vi "Drive Controller.vi"(8 "error in":errorcluster) -> ()   [LabVIEW 2017]
doc: "This VI executes continuously carrying out the current operation and responding to updates or new operation requests. It will often contain the timing or control code that is difficult to place directly in TeleOp. This VI generally opens all sensors and motors and isolates the rest of the robot code from knowing implementation details of how the operations are carried out."
uses:
  <vilib>/Rock Robotics/WPI/Framework/Completion Status.ctl
  Drive Setpoints.ctl
  Drive Operations.ctl
  <vilib>/Rock Robotics/WPI/SafetyOutput/WPI_SafetyOutputConfigMenu.ctl
  Phoenix-LabVIEW/Motor Controller/Controls/CTRE_Phoenix_MotorControl_FeedbackDevice.ctl
  Phoenix-LabVIEW/Motor Controller/Controls/CTRE_Phoenix_MotorControl_NeutralMode.ctl
  Drive Published Globals.vi
  <vilib>/Rock Robotics/WPI/RobotDrive/WPI_RobotDriveOpen2MotorWithExistingMotors.vi
  Framework/Robot Global Data.vi
  Phoenix-LabVIEW/Motor Controller/Get/CTRE_Phoenix_MotorController_GetQuadratureData.vi
  <vilib>/Rock Robotics/WPI/RobotDrive/WPI_RobotDriveArcadeDrive_Standard(NoSaturation).vi
  <vilib>/Rock Robotics/Network Tables/NT Write Numeric Array.vi
panel:
  out "RDriveEncoder 2":i32
  out "LDriveEncoder 2":i32
  out "UseLDriveEncoder 2":bool
  out "TargetEncValue":dbl
  out "DegreesToTravel":dbl
  out "UseLDriveEncoder":bool
  out "LDriveEncoder":i32
  out "RDriveEncoder":i32
  out "DriveLastCommandStatus":T1
  in  "Interactive Values":T2
  in  "Buttons":cluster{"Execute Cmd":bool, "Abort Cmd":bool}
  out "Command Timing":cluster{"Start Time (ms)":u32, "Iterations":i32}
  out "Status":T1
  out "Setpoints":T4(graph)
  out "Current\nCmd":string
  # "Tip: The graph shows the motor setpoints. It may also be helpful to observe inputs and sensor values.  You may also want to display tuning or debugging controls."
  # "Interactive Command: You may fill in the settings for a command\nand schedule it with the Execute button. You can observe and abort\nany command while fine tuning the code for the controller."
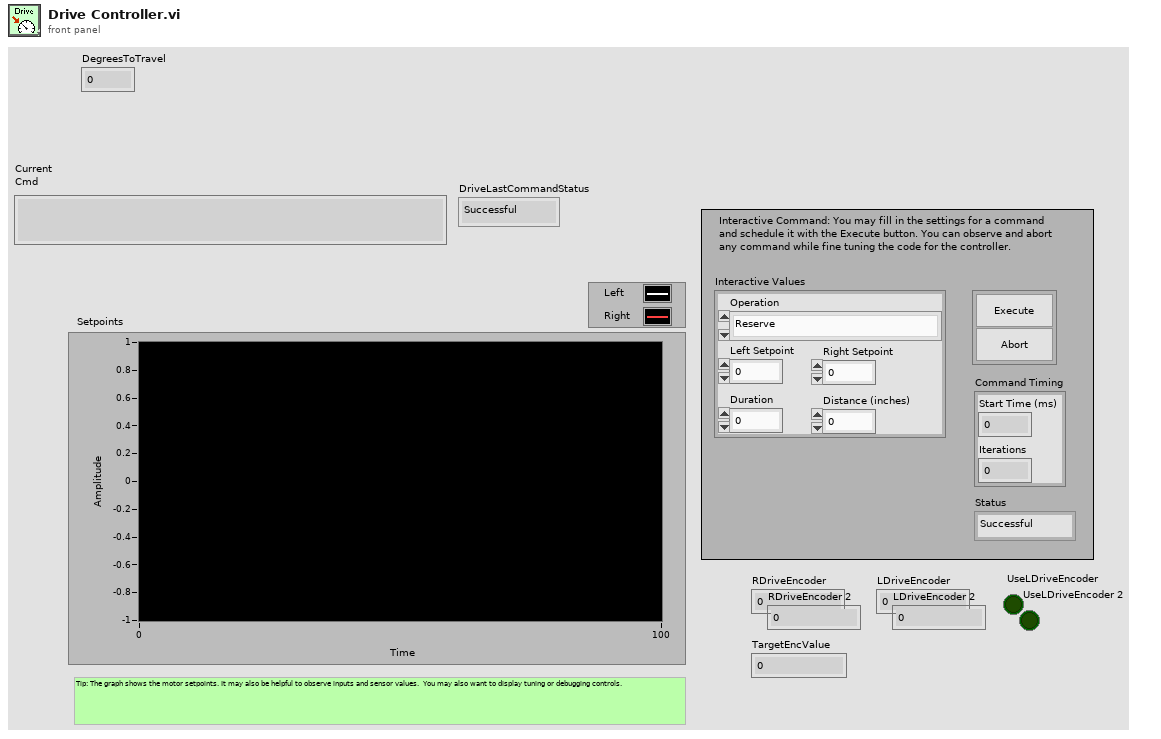
[diagram p1: front panel]
types:
  T1 = typedef "Completion Status.ctl" = enum16{"Successful", "Aborted", "Incomplete"}
  T2 = typedef "Drive Setpoints.ctl" = cluster{"Operation":T3, "Left Setpoint":dbl, "Right Setpoint":dbl, "Duration":dbl, "Distance (inches)":dbl}
  T3 = typedef "Drive Operations.ctl" = enum16{"Reserve", "Read Current", "Immediate", "Drive for Time", "Drive for Distance", "Rotate"}
  T4 = cluster{"Left Setpoint":dbl, "Right Setpoint":dbl}
  T5 = typedef "WPI_SafetyOutputConfigMenu.ctl" = enum16{"Enable", "Disable"}
  T6 = typedef "CTRE_Phoenix_MotorControl_FeedbackDevice.ctl" = i8
  T7 = typedef "WPI_MotorControlDeviceRef.ctl" = cluster{"DeviceStatus":errorcluster, "Type":T8, "PWM":cluster{"PWM Channel":T9, "DeadBand":T10}, "CAN":cluster{"Device Number":u8, "SetOutput VI Ref":variant, "GetOutput VI Ref":variant, "Enable VI Ref":variant, "Disable VI Ref":variant, "Data":variant}, "Invert":bool, "DIO PWM":cluster{"PWM \"Enable\" Channel":T9, "DIOChannel":T11, "PWM Rate":dbl}}
  T8 = typedef "WPI_MotorControlType.ctl" = enum16{"PWM", "CAN", "DIO PWM"}
  T9 = typedef "FPGA_DIOPWMChannel.ctl" = enum8{"PWM 0", "PWM 1", "PWM 2", "PWM 3", "PWM 4", "PWM 5", "PWM 6", "PWM 7", "PWM 8", "PWM 9", "PWM MXP 0", "PWM MXP 1", "PWM MXP 2", "PWM MXP 3", "PWM MXP 4", "PWM MXP 5", "PWM MXP 6", "PWM MXP 7", "PWM MXP 8", "PWM MXP 9", "Invalid"}
  T10 = typedef "WPI_PWMDeadband.ctl" = cluster{"Name":string, "maxPositivePwm":i32, "minPositivePwm":i32, "centerPwm":i32, "maxNegativePwm":i32, "minNegativePwm":i32, "angularRange":u16}
  T11 = typedef "FPGA_DIOChannel.ctl" = enum8{"DIO 0", "DIO 1", "DIO 2", "DIO 3", "DIO 4", "DIO 5", "DIO 6", "DIO 7", "DIO 8", "DIO 9", "DIO MXP 0", "DIO MXP 1", "DIO MXP 2", "DIO MXP 3", "DIO MXP 4", "DIO MXP 5", "DIO MXP 6", "DIO MXP 7", "DIO MXP 8", "DIO MXP 9", "DIO MXP 10", "DIO MXP 11", "DIO MXP 12", "DIO MXP 13", "DIO MXP 14", "DIO MXP 15", "SPI Port CS1", "SPI Port CS2", "SPI Port CS3", "SPI Port MISO", "SPI Port MOSI", "Invalid"}
  T12 = typedef "WPI_RobotDriveDevRef.ctl" = cluster{"DevStatus":errorcluster, "Motors[]":T7[], "Square Inputs":bool, "Max Output":dbl}
  T13 = typedef "Command Status Info.ctl" = cluster{"Name":string, "Status":T1, "notifier out":T14}
  T14 = typedef "Completion Notifier.ctl" = refnum<notifier>
  T15 = cluster{"SubSystem Data":T2, cluster{"Start Time (ms)":u32, "Iterations":i32}, cluster{"Command Info":T13, "Description":string, "Default Command":T2, "queue out":refnum<queue>, "Subsystem Name":string}}
  T16 = typedef "CTRE_Phoenix_MotorControl_NeutralMode.ctl" = enum8{"EEPROMSetting", "Override to Coast", "Override to Brake"}
  T17 = cluster{"SubSystem Data":T2, cluster{"Start Time (ms)":u32, "Iterations":i32}, "Default Command Arguments":cluster{"Command Info":T13, "Description":string, "Default Command":T2, "queue out":refnum<queue>, "Subsystem Name":string}}
  T18 = cluster{"Don't move motors while reserved":dbl, "Don't move motors while reserved":dbl}
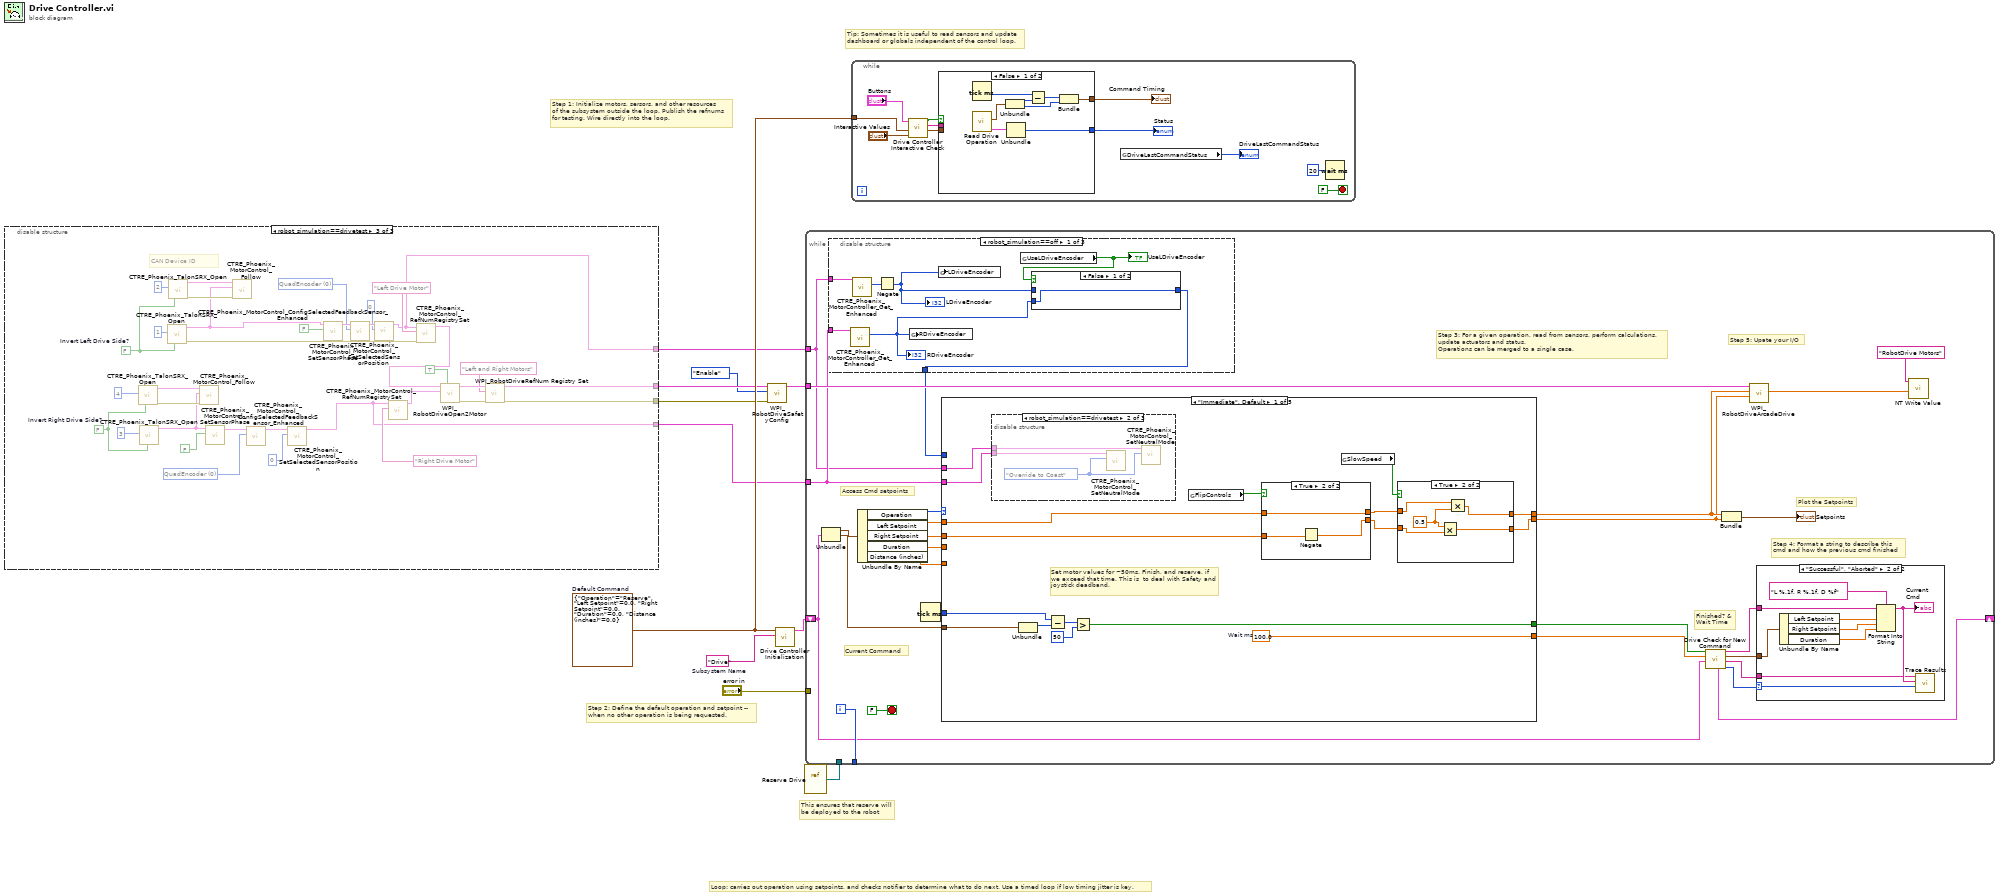
[diagram p0: block diagram]
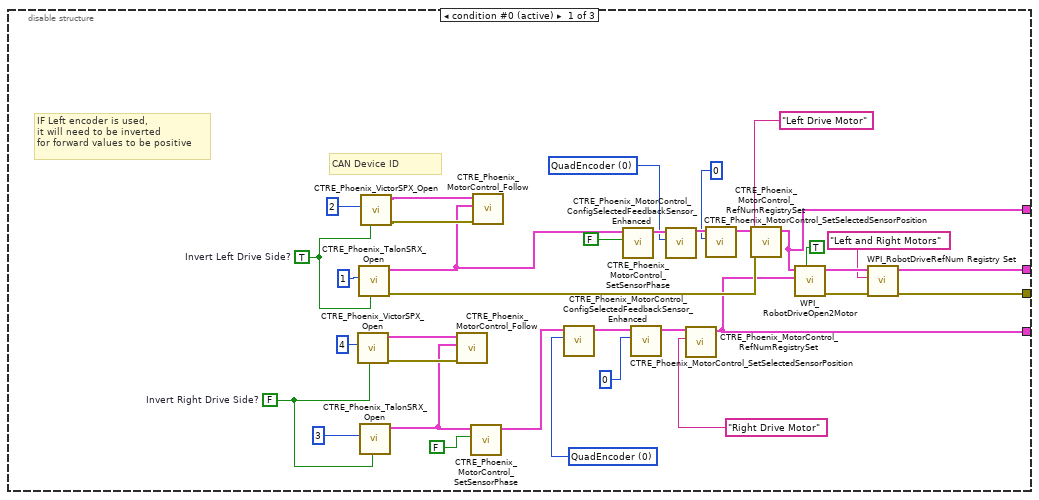
[diagram p2: hidden frame]
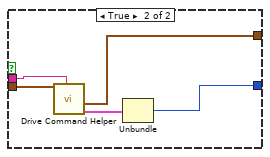
[diagram p4: hidden frame]
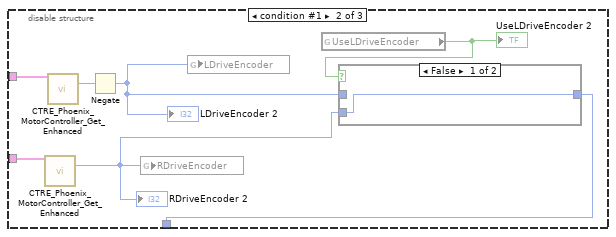
[diagram p6: hidden frame]
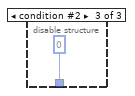
[diagram p8: hidden frame]
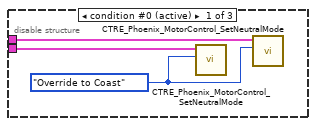
[diagram p11: hidden frame]
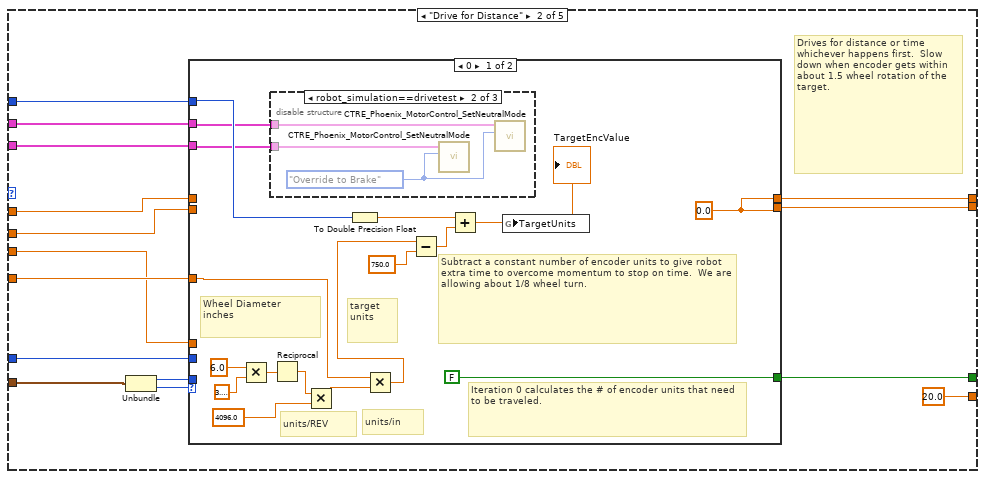
[diagram p14: hidden frame]
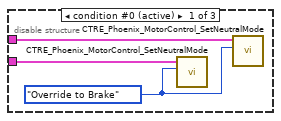
[diagram p15: hidden frame]
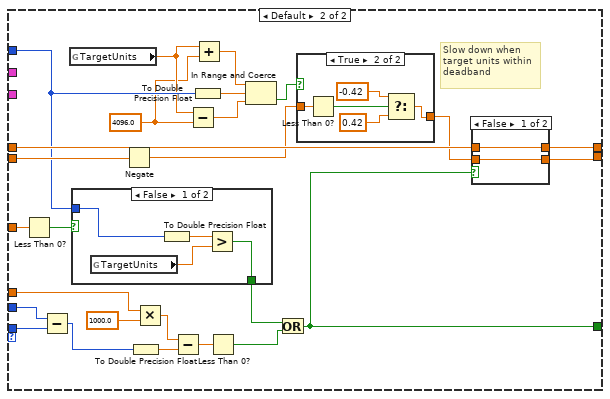
[diagram p17: hidden frame]
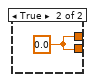
[diagram p19: hidden frame]
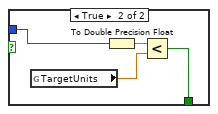
[diagram p20: hidden frame]
diagram:
  w6 = T2 {"Operation"=enum."Reserve", "Left Setpoint"=0.0, "Right Setpoint"=0.0, "Duration"=0.0, "Distance (inches)"=0.0}  # Default Command
  w11 = "Drive"  # Subsystem Name
  # "This ensures that reserve will\nbe deployed to the robot"
  # "Tip: Sometimes it is useful to read sensors and update\ndashboard or globals independent of the control loop."
  # "Step 2: Define the default operation and setpoint --\nwhen no other operation is being requested."
  # "Step 1: Initialize motors, sersors, and other resources\nof the subsystem outside the loop. Publish the refnums\nfor testing. Wire directly into the loop."
  # "Loop: carries out operation using setpoints, and checks notifier to determine what to do next. Use a timed loop if low timing jitter is key."
  n1 = disable-structure shown="robot_simulation==drivetest" {
    disable-tunnel: [w39 _ w64] -> w5
    disable-tunnel: [w38 _ w63] -> w4
    disable-tunnel: [w21 _ w49] -> w2
    disable-tunnel: [w15 _ w50] -> w1
    frame condition #0 (active) {
      w17 = T6 0 items=["None"=-1, "QuadEncoder"=0, "Analog"=2, "Tachometer"=4, "Pulse Width Encoded Position"=8, "Sensor Sum (S0 + S1)"=9, "Sensor Difference (D0 - D1)"=10, "Remote Source 0"=11, "Remote Source 1"=12, "Software Emulated"=15] ("Feedback Device")
      w26 = T6 0 items=["None"=-1, "QuadEncoder"=0, "Analog"=2, "Tachometer"=4, "Pulse Width Encoded Position"=8, "Sensor Sum (S0 + S1)"=9, "Sensor Difference (D0 - D1)"=10, "Remote Source 0"=11, "Remote Source 1"=12, "Software Emulated"=15] ("Feedback Device")
      w32 = TRUE  # Invert Left Drive Side?
      w30 = FALSE  # Invert Right Drive Side?
      # "IF Left encoder is used,\nit will need to be inverted\nfor forward values to be positive"
      # "CAN Device ID"
      n2 = call "CTRE_Phoenix_VictorSPX_Open.vi"("Invert"=w30, "Device Number"=u8 4) -> ("error out"=w41:errorcluster, "CAN Talon SRX Ref"=w40:T7)  [unwired: 8 in]
      n3 = call "CTRE_Phoenix_TalonSRX_Open.vi"("Invert"=w32, "Device Number"=u8 1) -> ("error out"=w42:errorcluster, "CAN Talon SRX Ref"=w13:T7)  [unwired: 8 in]
      n4 = call "CTRE_Phoenix_TalonSRX_Open.vi"("Invert"=w30, "Device Number"=u8 3) -> ("CAN Talon SRX Ref"=w28:T7)  [unwired: 8 in, 1 out]
      n5 = call "CTRE_Phoenix_VictorSPX_Open.vi"("Invert"=w32, "Device Number"=u8 2) -> ("error out"=w35:errorcluster, "CAN Talon SRX Ref"=w36:T7)  [unwired: 8 in]
      n6 = call "CTRE_Phoenix_MotorControl_Follow.vi"("error in (no error)"=w41, "Master Controller to Follow"=w28, "PhoenixMotorControlDevRef"=w40) -> ()  [unwired: 7 in, 2 out]
      n7 = call "CTRE_Phoenix_MotorControl_SetSensorPhase.vi"("PhaseSensor"=FALSE, "PhoenixMotorControlDevRef"=w28) -> ("PhoenixMotorControlDevRef"=w24:T7)  [unwired: 8 in, 1 out]
      n8 = call "CTRE_Phoenix_MotorControl_Follow.vi"("error in (no error)"=w35, "Master Controller to Follow"=w13, "PhoenixMotorControlDevRef"=w36) -> ()  [unwired: 7 in, 2 out]
      n9 = call "CTRE_Phoenix_MotorControl_ConfigSelectedFeedbackSensor_Enhanced.vi"("Feedback Device"=w26, "PhoenixMotorControlDevRef"=w24) -> ("PhoenixMotorControlDevRef"=w23:T7)  [unwired: 8 in, 1 out]
      n10 = call "CTRE_Phoenix_MotorControl_SetSensorPhase.vi"("PhaseSensor"=FALSE, "PhoenixMotorControlDevRef"=w13) -> ("PhoenixMotorControlDevRef"=w19:T7)  [unwired: 8 in, 1 out]
      n11 = call "CTRE_Phoenix_MotorControl_SetSelectedSensorPosition.vi"("New Sensor Position"=0, "PhoenixMotorControlDevRef"=w23) -> ("PhoenixMotorControlDevRef"=w22:T7)  [unwired: 8 in, 1 out]
      n12 = call "CTRE_Phoenix_MotorControl_ConfigSelectedFeedbackSensor_Enhanced.vi"("Feedback Device"=w17, "PhoenixMotorControlDevRef"=w19) -> ("PhoenixMotorControlDevRef"=w20:T7)  [unwired: 8 in, 1 out]
      n13 = call "CTRE_Phoenix_MotorControl_RefNumRegistrySet.vi"("refnum name"="Right Drive Motor", "PhoenixMotorControlDevRef"=w22) -> ("PhoenixMotorControlDevRef"=w21:T7)  [unwired: 8 in, 1 out]
      n14 = call "CTRE_Phoenix_MotorControl_SetSelectedSensorPosition.vi"("New Sensor Position"=0, "PhoenixMotorControlDevRef"=w20) -> ("PhoenixMotorControlDevRef"=w14:T7)  [unwired: 8 in, 1 out]
      n15 = call "CTRE_Phoenix_MotorControl_RefNumRegistrySet.vi"("error in (no error)"=w42, "refnum name"="Left Drive Motor", "PhoenixMotorControlDevRef"=w14) -> ("PhoenixMotorControlDevRef"=w15:T7)  [unwired: 7 in, 1 out]
      n16 = call-poly <vilib>:"WPI_RobotDriveOpen2Motor.vi"("Square Inputs"=TRUE, "Right Motor Dev Ref"=w21, "Left Motor Dev Ref"=w15) -> ("error out"=w44:errorcluster, "RobotDriveDevRef"=w46:T12)  [unwired: 2 in, 5 out]
      n17 = call <vilib>:"WPI_RobotDriveRefNum Registry Set.vi"("error in (no error)"=w44, "refnum name"="Left and Right Motors", "RobotDriveDevRef"=w46) -> ("error out"=w38:errorcluster, "RobotDriveDevRef"=w39:T12)  [unwired: 1 in, 6 out]
    }
    frame condition #1 {
    }
    frame condition #2 {
      w52 = T6 0 items=["None"=-1, "QuadEncoder"=0, "Analog"=2, "Tachometer"=4, "Pulse Width Encoded Position"=8, "Sensor Sum (S0 + S1)"=9, "Sensor Difference (D0 - D1)"=10, "Remote Source 0"=11, "Remote Source 1"=12, "Software Emulated"=15] ("Feedback Device")
      w56 = T6 0 items=["None"=-1, "QuadEncoder"=0, "Analog"=2, "Tachometer"=4, "Pulse Width Encoded Position"=8, "Sensor Sum (S0 + S1)"=9, "Sensor Difference (D0 - D1)"=10, "Remote Source 0"=11, "Remote Source 1"=12, "Software Emulated"=15] ("Feedback Device")
      w71 = FALSE  # Invert Left Drive Side?
      w62 = FALSE  # Invert Right Drive Side?
      # "CAN Device ID"
      n18 = call "CTRE_Phoenix_TalonSRX_Open.vi"("Invert"=w62, "Device Number"=u8 4) -> ("error out"=w74:errorcluster, "CAN Talon SRX Ref"=w73:T7)  [unwired: 8 in]
      n19 = call "CTRE_Phoenix_TalonSRX_Open.vi"("Invert"=w62, "Device Number"=u8 3) -> ("CAN Talon SRX Ref"=w61:T7)  [unwired: 8 in, 1 out]
      n20 = call "CTRE_Phoenix_TalonSRX_Open.vi"("Invert"=w71, "Device Number"=u8 1) -> ("error out"=w76:errorcluster, "CAN Talon SRX Ref"=w48:T7)  [unwired: 8 in]
      n21 = call "CTRE_Phoenix_TalonSRX_Open.vi"("Invert"=w71, "Device Number"=u8 2) -> ("error out"=w68:errorcluster, "CAN Talon SRX Ref"=w69:T7)  [unwired: 8 in]
      n22 = call "CTRE_Phoenix_MotorControl_Follow.vi"("error in (no error)"=w74, "Master Controller to Follow"=w61, "PhoenixMotorControlDevRef"=w73) -> ()  [unwired: 7 in, 2 out]
      n23 = call "CTRE_Phoenix_MotorControl_SetSensorPhase.vi"("PhaseSensor"=FALSE, "PhoenixMotorControlDevRef"=w61) -> ("PhoenixMotorControlDevRef"=w58:T7)  [unwired: 8 in, 1 out]
      n24 = call "CTRE_Phoenix_MotorControl_Follow.vi"("error in (no error)"=w68, "Master Controller to Follow"=w48, "PhoenixMotorControlDevRef"=w69) -> ()  [unwired: 7 in, 2 out]
      n25 = call "CTRE_Phoenix_MotorControl_ConfigSelectedFeedbackSensor_Enhanced.vi"("Feedback Device"=w56, "PhoenixMotorControlDevRef"=w58) -> ("PhoenixMotorControlDevRef"=w59:T7)  [unwired: 8 in, 1 out]
      n26 = call "CTRE_Phoenix_MotorControl_SetSelectedSensorPosition.vi"("New Sensor Position"=0, "PhoenixMotorControlDevRef"=w59) -> ("PhoenixMotorControlDevRef"=w49:T7)  [unwired: 8 in, 1 out]
      n27 = call "CTRE_Phoenix_MotorControl_SetSensorPhase.vi"("PhaseSensor"=FALSE, "PhoenixMotorControlDevRef"=w48) -> ("PhoenixMotorControlDevRef"=w54:T7)  [unwired: 8 in, 1 out]
      n28 = call "CTRE_Phoenix_MotorControl_ConfigSelectedFeedbackSensor_Enhanced.vi"("Feedback Device"=w52, "PhoenixMotorControlDevRef"=w54) -> ("PhoenixMotorControlDevRef"=w55:T7)  [unwired: 8 in, 1 out]
      n29 = call "CTRE_Phoenix_MotorControl_SetSelectedSensorPosition.vi"("New Sensor Position"=0, "PhoenixMotorControlDevRef"=w55) -> ("PhoenixMotorControlDevRef"=w50:T7)  [unwired: 8 in, 1 out]
      n30 = call "CTRE_Phoenix_MotorControl_RefNumRegistrySet.vi"("refnum name"="Right Drive Motor", "PhoenixMotorControlDevRef"=w49) -> ("PhoenixMotorControlDevRef"=w66:T7)  [unwired: 8 in, 1 out]
      n31 = call "CTRE_Phoenix_MotorControl_RefNumRegistrySet.vi"("error in (no error)"=w76, "refnum name"="Left Drive Motor", "PhoenixMotorControlDevRef"=w50) -> ("PhoenixMotorControlDevRef"=w65:T7)  [unwired: 7 in, 1 out]
      n32 = call-poly <vilib>:"WPI_RobotDriveOpen2Motor.vi"("Square Inputs"=TRUE, "Right Motor Dev Ref"=w66, "Left Motor Dev Ref"=w65) -> ("error out"=w79:errorcluster, "RobotDriveDevRef"=w81:T12)  [unwired: 2 in, 5 out]
      n33 = call <vilib>:"WPI_RobotDriveRefNum Registry Set.vi"("error in (no error)"=w79, "refnum name"="Left and Right Motors", "RobotDriveDevRef"=w81) -> ("error out"=w63:errorcluster, "RobotDriveDevRef"=w64:T12)  [unwired: 1 in, 6 out]
    }
  }
  n34 = call <vilib>:"WPI_RobotDriveSafetyConfig.vi"("error in (no error)"=w4, "mode"=WPI_SafetyOutputConfigMenu."Enable", "RobotDriveDevRef"=w5) -> ("RobotDriveDevRef"=w10:T12)  [unwired: 7 in, 1 out]
  n35 = call "Drive Controller Initialization.vi"("Subsystem Name"=w11, "Default Command"=w6) -> ("Current Command"=w8:T15)  [unwired: 9 in]
  n36 = vi-ref "Reserve Drive.vi"() -> (w7:refnum<vi>)
  n37 = while {
    shift-right: [w96] -> _
    shift-left: w8 -> [w91]
    tunnel: [w107] -> _
    tunnel: w10 -> [w87]
    tunnel: "error in" -> [_]
    tunnel: w7 -> [_]
    tunnel: w2 -> [w85]
    tunnel: w1 -> [w82]
    i -> [w107]
    stop <- FALSE stop-if-true
    # "Step 5: Upate your I/O"
    # "Step 4: Format a string to describe this\ncmd and how the previous cmd finished"
    # "Current Command"
    # "Plot the Setpoints"
    # "Access Cmd setpoints"
    # "Finished? &\nWait Time"
    # "Step 3: For a given operation, read from sensors, perform calculations,\nupdate actuators and status.\nOperations can be merged to a single case."
    n38 = Unbundle(w91) -> ("SubSystem Data"=w103:T2, w92:cluster{"Start Time (ms)":u32, "Iterations":i32})  [unwired: 1 out]
    n39 = disable-structure shown="robot_simulation==off" {
      disable-tunnel: [w114 w123 0 ("Quadrature Position")] -> w86
      disable-tunnel: w85 -> [w110 w119 _]
      disable-tunnel: w82 -> [w109 w118 _]
      frame condition #0 (active) {
        n40 = call-poly "CTRE_Phoenix_MotorController_Get_Enhanced.vi"("PhoenixMotorControlDevRef"=w110) -> ("Quadrature Position"=w115:i32)  [unwired: 11 in, 3 out]
        "RDriveEncoder" <- w115
        n41 = call-poly "CTRE_Phoenix_MotorController_Get_Enhanced.vi"("PhoenixMotorControlDevRef"=w109) -> ("Quadrature Position"=w112:i32)  [unwired: 11 in, 3 out]
        n42 = Negate(x=w112) -> (-x=w111:i32)
        "LDriveEncoder" <- w111
        n43 = global write "Robot Global Data.vi" "RDriveEncoder"(w115) -> ()
        n44 = global write "Robot Global Data.vi" "LDriveEncoder"(w111) -> ()
        n45 = global read "Robot Global Data.vi" "UseLDriveEncoder"() -> (w113:bool)
        "UseLDriveEncoder" <- w113
        n46 = case shown="False" w113 {
          tunnel: [w116 w117] -> w114
          tunnel: w111 -> [_ w117]
          tunnel: w115 -> [w116 _]
          frame False {
          }
          frame True {
          }
        }
      }
      frame condition #1 {
        n47 = call-poly "CTRE_Phoenix_MotorController_Get_Enhanced.vi"("PhoenixMotorControlDevRef"=w119) -> ("Quadrature Position"=w124:i32)  [unwired: 11 in, 3 out]
        "RDriveEncoder 2" <- w124
        n48 = call-poly "CTRE_Phoenix_MotorController_Get_Enhanced.vi"("PhoenixMotorControlDevRef"=w118) -> ("Quadrature Position"=w121:i32)  [unwired: 11 in, 3 out]
        n49 = Negate(x=w121) -> (-x=w120:i32)
        "LDriveEncoder 2" <- w120
        n50 = global write "Robot Global Data.vi" "RDriveEncoder"(w124) -> ()
        n51 = global write "Robot Global Data.vi" "LDriveEncoder"(w120) -> ()
        n52 = global read "Robot Global Data.vi" "UseLDriveEncoder"() -> (w122:bool)
        "UseLDriveEncoder 2" <- w122
        n53 = case shown="False" w122 {
          tunnel: [w125 w126] -> w123
          tunnel: w120 -> [_ w126]
          tunnel: w124 -> [w125 _]
          frame False {
          }
          frame True {
          }
        }
      }
      frame condition #2 {
      }
    }
    n54 = Unbundle By Name(w103) -> ("Operation"=w102:T3, "Left Setpoint"=w101:dbl, "Right Setpoint"=w100:dbl, "Duration"=w99:dbl, "Distance (inches)"=w88:dbl)
    n55 = Tick Count (ms)() -> (millisecond timer value=w98:u32)
    n56 = case shown="\"Immediate\", Default" w102 {
      tunnel: [w153 20.0 ("Infinite") 50.0 ("y") w294 250.0 ("Infinite")] -> w83
      tunnel: [w148 w183 w253 w300 FALSE ("ignore previous (F)")] -> w84
      tunnel: w92 -> [w147 w186 w258 w302 _]
      tunnel: [w137 w178 w255 w299 w312] -> w105
      tunnel: [w138 w177 0.0 ("Don't move motors while reserved") w291 w312] -> w104
      tunnel: w101 -> [w146 w175 w260 w299 _]
      tunnel: w100 -> [w145 w176 w259 w290 _]
      tunnel: w99 -> [_ w179 _ w298 _]
      tunnel: w98 -> [w149 w180 _ w297 _]
      tunnel: w88 -> [_ w184 _ _ _]
      tunnel: w86 -> [_ w174 _ _ _]
      tunnel: w85 -> [w144 w172 _ w292 w313]
      tunnel: w82 -> [w143 w173 _ w293 w314]
      frame "Immediate", Default {
        w153 = 100.0  # Wait ms
        # "Set motor values for ~50ms. Finish, and reserve, if\nwe exceed that time. This is  to deal with Safety and\njoystick deadband."
        n57 = disable-structure shown="robot_simulation==drivetest" {
          disable-tunnel: w144 -> [w163 w166 _]
          disable-tunnel: w143 -> [w162 w165 _]
          frame condition #0 (active) {
            w161 = CTRE_Phoenix_MotorControl_NeutralMode."Override to Coast" ("Motor Control Neutral Mode")
            n58 = call "CTRE_Phoenix_MotorControl_SetNeutralMode.vi"("Motor Control Neutral Mode"=w161, "PhoenixMotorControlDevRef"=w163) -> ()  [unwired: 8 in, 2 out]
            n59 = call "CTRE_Phoenix_MotorControl_SetNeutralMode.vi"("Motor Control Neutral Mode"=w161, "PhoenixMotorControlDevRef"=w162) -> ()  [unwired: 8 in, 2 out]
          }
          frame condition #1 {
            w164 = CTRE_Phoenix_MotorControl_NeutralMode."Override to Coast" ("Motor Control Neutral Mode")
            n60 = call "CTRE_Phoenix_MotorControl_SetNeutralMode.vi"("Motor Control Neutral Mode"=w164, "PhoenixMotorControlDevRef"=w166) -> ()  [unwired: 8 in, 2 out]
            n61 = call "CTRE_Phoenix_MotorControl_SetNeutralMode.vi"("Motor Control Neutral Mode"=w164, "PhoenixMotorControlDevRef"=w165) -> ()  [unwired: 8 in, 2 out]
          }
          frame condition #2 {
          }
        }
        n62 = Unbundle(w147) -> ("Start Time (ms)"=w150:u32)  [unwired: 1 out]
        n63 = Subtract(x=w149, y=w150) -> (x-y=w151:u32)
        n64 = Greater?(x=w151, y=u8 50 ("Left Motor")) -> (0:w148:bool)
        n65 = global read "Robot Global Data.vi" "FlipControls"() -> (w142:bool)
        n66 = case shown="True" w142 {
          tunnel: w146 -> [w168 w169]
          tunnel: w145 -> [w167 w171]
          tunnel: [w168 w169] -> w139
          tunnel: [w167 w170] -> w140
          frame False {
          }
          frame True {
            n67 = Negate(x=w171) -> (-x=w170:dbl)
          }
        }
        n68 = global read "Robot Global Data.vi" "SlowSpeed"() -> (w141:bool)
        n69 = case shown="True" w141 {
          tunnel: w140 -> [w154 w160]
          tunnel: w139 -> [w155 w158]
          tunnel: [w154 w159] -> w138
          tunnel: [w155 w157] -> w137
          frame False {
          }
          frame True {
            w156 = 0.5 ("x")
            n70 = Multiply(x=w156, y=w160) -> (x*y=w159:dbl)
            n71 = Multiply(x=w158, y=w156) -> (x*y=w157:dbl)
          }
        }
      }
      frame "Drive for Distance" {
        # "Drives for distance or time whichever happens first.  Slow down when encoder gets within about 1.5 wheel rotation of the target."
        n72 = Unbundle(w186) -> ("Start Time (ms)"=w181:u32, "Iterations"=w185:i32)
        n73 = case shown="0" w185 {
          tunnel: w184 -> [w201 w235]
          tunnel: w174 -> [w196 w218]
          tunnel: [FALSE w221] -> w183
          tunnel: w181 -> [_ w233]
          tunnel: w180 -> [_ w232]
          tunnel: w179 -> [_ w230]
          tunnel: [w191 w224] -> w178
          tunnel: w176 -> [_ w220]
          tunnel: [w191 w222] -> w177
          tunnel: w175 -> [_ w223]
          tunnel: w173 -> [w192 _]
          tunnel: w172 -> [w193 _]
          frame 0 {
            w191 = 0.0 ("Left Setpoint")
            # "Subtract a constant number of encoder units to give robot extra time to overcome momentum to stop on time.  We are allowing about 1/8 wheel turn."
            # "Iteration 0 calculates the # of encoder units that need to be traveled."
            # "target\nunits"
            # "units/in"
            # "units/REV"
            # "Wheel Diameter \ninches"
            n74 = Multiply(x=6.0, y=3.141592653589793) -> (x*y=w199:dbl)
            n75 = disable-structure shown="robot_simulation==drivetest" {
              disable-tunnel: w193 -> [w205 w208 _]
              disable-tunnel: w192 -> [w204 w207 _]
              frame condition #0 (active) {
                w206 = CTRE_Phoenix_MotorControl_NeutralMode."Override to Brake" ("Motor Control Neutral Mode")
                n76 = call "CTRE_Phoenix_MotorControl_SetNeutralMode.vi"("Motor Control Neutral Mode"=w206, "PhoenixMotorControlDevRef"=w205) -> ()  [unwired: 8 in, 2 out]
                n77 = call "CTRE_Phoenix_MotorControl_SetNeutralMode.vi"("Motor Control Neutral Mode"=w206, "PhoenixMotorControlDevRef"=w204) -> ()  [unwired: 8 in, 2 out]
              }
              frame condition #1 {
                w209 = CTRE_Phoenix_MotorControl_NeutralMode."Override to Brake" ("Motor Control Neutral Mode")
                n78 = call "CTRE_Phoenix_MotorControl_SetNeutralMode.vi"("Motor Control Neutral Mode"=w209, "PhoenixMotorControlDevRef"=w208) -> ()  [unwired: 8 in, 2 out]
                n79 = call "CTRE_Phoenix_MotorControl_SetNeutralMode.vi"("Motor Control Neutral Mode"=w209, "PhoenixMotorControlDevRef"=w207) -> ()  [unwired: 8 in, 2 out]
              }
              frame condition #2 {
              }
            }
            n80 = Reciprocal(x=w199) -> (1/x=w198:dbl)
            n81 = Multiply(x=w198, y=4096.0 ("x")) -> (x*y=w200:dbl)
            n82 = To Double Precision Float(number=w196) -> (double precision float=w190:dbl)
            n83 = Multiply(x=w201, y=w200) -> (x*y=w188:dbl)
            n84 = Subtract(x=w188, y=750.0) -> (x-y=w189:dbl)
            n85 = Add(x=w190, y=w189) -> (x+y=w195:dbl)
            "TargetEncValue" <- w195
            n86 = global write "Drive Published Globals.vi" "TargetUnits"(w195) -> ()
          }
          frame Default {
            w216 = 4096.0 ("y")
            # "Slow down when\ntarget units within\ndeadband"
            n87 = Less Than 0?(x=w235) -> (x < 0?=w234:bool)
            n88 = Subtract(x=w232, y=w233) -> (x-y=w228:u32)
            n89 = global read "Drive Published Globals.vi" "TargetUnits"() -> (w217:dbl)
            n90 = case shown="False" w234 {
              tunnel: w218 -> [w247 w251]
              tunnel: [w246 w250] -> w226
              frame False {
                n91 = global read "Drive Published Globals.vi" "TargetUnits"() -> (w248:dbl)
                n92 = To Double Precision Float(number=w247) -> (double precision float=w245:dbl)
                n93 = Greater?(x=w245, y=w248) -> (0:w246:bool)
              }
              frame True {
                n94 = global read "Drive Published Globals.vi" "TargetUnits"() -> (w252:dbl)
                n95 = To Double Precision Float(number=w251) -> (double precision float=w249:dbl)
                n96 = Less?(x=w249, y=w252) -> (x < y?=w250:bool)
              }
            }
            n97 = Negate(x=w220) -> (-x=w213:dbl)
            n98 = To Double Precision Float(number=w228) -> (double precision float=w210:dbl)
            n99 = Multiply(x=w230, y=1000.0) -> (x*y=w229:dbl)
            n100 = Subtract(x=w229, y=w210) -> (x-y=w227:dbl)
            n101 = Subtract(x=w217, y=w216) -> (x-y=w214:dbl)
            n102 = To Double Precision Float(number=w218) -> (double precision float=w219:dbl)
            n103 = Add(x=w217, y=w216) -> (x+y=w215:dbl)
            n104 = Less Than 0?(x=w227) -> (x < 0?=w225:bool)
            n105 = In Range and Coerce(upper limit=w215, x=w219, lower limit=w214) -> (In Range?=w211:bool)  [unwired: 1 out]
            n106 = Or(x=w226, y=w225) -> (x .or. y?=w221:bool)
            n107 = case shown="True" w211 {
              tunnel: w213 -> [w236 w241]
              tunnel: [w236 w239] -> w212
              frame False {
              }
              frame True {
                n108 = Less Than 0?(x=w241) -> (x < 0?=w240:bool)
                n109 = Select(t=-0.42 ("f"), s=w240, f=0.42) -> (s? t:f=w239:dbl)
              }
            }
            n110 = case shown="False" w221 {
              tunnel: [w243 w244] -> w224
              tunnel: w223 -> [w243 _]
              tunnel: w212 -> [w242 _]
              tunnel: [w242 w244] -> w222
              frame False {
              }
              frame True {
                w244 = 0.0 ("Left Setpoint")
              }
            }
          }
        }
      }
      frame "Rotate" {
        # "lowest speed"
        # "Deadband"
        # "Do we have more to travel?\nIf so, keep moving."
        # "Run motor for 50ms"
        # "scale speed down if less than 30. \nIf not, set motor power to 0.5"
        # "Calculate degrees remaining"
        n111 = global read "Robot Global Data.vi" "GyroHeading"() -> (w273:dbl)
        n112 = Unbundle(w258) -> ()  [unwired: 2 out]
        n113 = case shown="1" w259 {
          tunnel: w260 -> [w276 w282]
          tunnel: w273 -> [w278 w285]
          tunnel: [w275 w288] -> w264
          frame -1, Default {
            # "Going Left?"
            n114 = Subtract(x=w278, y=w276) -> (x-y=w277:dbl)
            n115 = Subtract(x=360.0, y=w276) -> (x-y=w279:dbl)
            n116 = Greater Or Equal?(x=w276, y=w278) -> (x >= y?=w281:bool)
            n117 = Add(x=w279, y=w278) -> (x+y=w274:dbl)
            n118 = Select(t=w274, s=w281, f=w277) -> (s? t:f=w275:dbl)
          }
          frame 1 {
            # "Going right?"
            n119 = Greater Or Equal?(x=w282, y=w285) -> (x >= y?=w289:bool)
            n120 = Subtract(x=w282, y=w285) -> (x-y=w287:dbl)
            n121 = Subtract(x=360.0, y=w285) -> (x-y=w284:dbl)
            n122 = Add(x=w282, y=w284) -> (x+y=w283:dbl)
            n123 = Select(t=w287, s=w289, f=w283) -> (s? t:f=w288:dbl)
          }
        }
        "DegreesToTravel" <- w264
        n124 = Subtract(x=w264, y=5.0) -> (x-y=w263:dbl)
        n125 = Greater?(x=w263, y=0.0 ("x")) -> (0:w254:bool)
        n126 = Not(x=w254) -> (.not. x?=w253:bool)
        n127 = Less?(x=w264, y=45.0) -> (x < y?=w271:bool)
        n128 = Divide(x=w264, y=60.0) -> (x/y=w267:dbl)
        n129 = Max & Min(x=w267, y=0.5) -> (max(x,y)=w265:dbl)  [unwired: 1 out]
        n130 = Select(t=w265, s=w271, f=0.6) -> (s? t:f=w269:dbl)
        n131 = Multiply(x=w269, y=w259) -> (x*y=w255:dbl)
      }
      frame "Drive for Time" {
        # "How much longer?\nUpdate motors every 50ms to\nkeep Safety happy"
        n132 = disable-structure shown="robot_simulation==drivetest" {
          disable-tunnel: w293 -> [w307 w310 _]
          disable-tunnel: w292 -> [w306 w309 _]
          frame condition #0 (active) {
            w308 = CTRE_Phoenix_MotorControl_NeutralMode."Override to Brake" ("Motor Control Neutral Mode")
            n133 = call "CTRE_Phoenix_MotorControl_SetNeutralMode.vi"("Motor Control Neutral Mode"=w308, "PhoenixMotorControlDevRef"=w306) -> ()  [unwired: 8 in, 2 out]
            n134 = call "CTRE_Phoenix_MotorControl_SetNeutralMode.vi"("Motor Control Neutral Mode"=w308, "PhoenixMotorControlDevRef"=w307) -> ()  [unwired: 8 in, 2 out]
          }
          frame condition #1 {
            w311 = CTRE_Phoenix_MotorControl_NeutralMode."Override to Brake" ("Motor Control Neutral Mode")
            n135 = call "CTRE_Phoenix_MotorControl_SetNeutralMode.vi"("Motor Control Neutral Mode"=w311, "PhoenixMotorControlDevRef"=w309) -> ()  [unwired: 8 in, 2 out]
            n136 = call "CTRE_Phoenix_MotorControl_SetNeutralMode.vi"("Motor Control Neutral Mode"=w311, "PhoenixMotorControlDevRef"=w310) -> ()  [unwired: 8 in, 2 out]
          }
          frame condition #2 {
          }
        }
        n137 = Unbundle(w302) -> ("Start Time (ms)"=w301:u32)  [unwired: 1 out]
        n138 = Subtract(x=w297, y=w301) -> (x-y=w305:u32)
        n139 = Multiply(x=w298, y=1000.0) -> (x*y=w304:dbl)
        n140 = Subtract(x=w304, y=w305) -> (x-y=w296:dbl)
        n141 = Less Or Equal To 0?(x=w296) -> (x <= 0?=w300:bool)
        n142 = Max & Min(x=w296, y=50.0) -> (min(x,y)=w294:dbl)  [unwired: 1 out]
        n143 = Negate(x=w290) -> (-x=w291:dbl)
      }
      frame "Reserve" {
        w312 = 0.0  # Don't move motors while reserved
        (unwired) -1.0  # Infinite
        # "If loop needs to poll sensors or other\nvalues, use a timeout value. -1 waits for\nnext command to be sent."
        n144 = disable-structure shown="Disabled" {
          disable-tunnel: w314 -> [w318 _]
          disable-tunnel: w313 -> [w317 _]
          frame Disabled {
            w319 = CTRE_Phoenix_MotorControl_NeutralMode."Override to Coast" ("Motor Control Neutral Mode")
            n145 = call "CTRE_Phoenix_MotorControl_SetNeutralMode.vi"("Motor Control Neutral Mode"=w319, "PhoenixMotorControlDevRef"=w317) -> ()  [unwired: 8 in, 2 out]
            n146 = call "CTRE_Phoenix_MotorControl_SetNeutralMode.vi"("Motor Control Neutral Mode"=w319, "PhoenixMotorControlDevRef"=w318) -> ()  [unwired: 8 in, 2 out]
          }
          frame Enabled {
          }
        }
      }
    }
    n147 = call "Drive Check for New Command.vi"("input cluster"=w91, "Wait time (ms)"=w83, "Finished?"=w84) -> ("Completion"=w97:T1, "Subsystem Name"=w93:string, "Current Command"=w94:T2, "Initial Trace String"=w95:string, "Next Command"=w96:T17)  [unwired: 4 in]
    n148 = Bundle("Don't move motors while reserved"=w105, "Don't move motors while reserved"=w104) -> (→"Setpoints":T18)  [unwired: 1 in]
    n149 = call-poly <vilib>:"WPI_RobotDriveArcadeDrive.vi"("Y axis value"=w104, "X axis value"=w105, "RobotDriveDevRef"=w87) -> ("Motor Values"=w89:dbl[])  [unwired: 6 in, 2 out]
    n150 = case shown="\"Successful\", \"Aborted\"" w97 {
      selector: w97 -> [_ w136]
      tunnel: w95 -> [_ w131]
      tunnel: w94 -> [_ w132]
      tunnel: w93 -> [_ w128]
      frame "Incomplete", Default {
        # "Continuing current command"
      }
      frame "Successful", "Aborted" {
        # "Report and setup for next command"
        n151 = Unbundle By Name(w132) -> ("Left Setpoint"=w134:dbl, "Right Setpoint"=w135:dbl, "Duration"=w129:dbl)
        n152 = Format Into String(format string="L %.1f, R %.1f, D %f", initial string=w131, w134, w135, w129) -> (resulting string=w130:string)  [unwired: 1 in, 1 out]
        "Current\nCmd" <- w130
        n153 = call <vilib>:"Trace Results.vi"("Status of previous command"=w136, "Description"=w130, "Subsystem"=w128) -> ()  [unwired: 9 in]
      }
    }
    n154 = call-poly <vilib>:"NT Write Value.vi"("Numeric Array"=w89, "Name"="RobotDrive Motors") -> ()  [unwired: 9 in, 1 out]
  }
  n155 = while {
    tunnel: w6 -> [w322]
    stop <- FALSE stop-if-true
    n156 = call "Drive Controller Interactive Check.vi"("Interactive Command In"="Interactive Values", "Default Command"=w322, "Buttons"="Buttons") -> ("Interactive Command Out"=w324:T2, "Trace String"=w325:string, "Schedule"=w326:bool)  [unwired: 6 in]
    n157 = case shown="False" w326 {
      tunnel: [w335 w343] -> w327
      tunnel: [w334 w339] -> w328
      tunnel: w325 -> [_ w341]
      tunnel: w324 -> [_ w340]
      frame False {
        n158 = Tick Count (ms)() -> (millisecond timer value=w338:u32)
        n159 = call "Read Drive Operation.vi"() -> ("Command Info"=w332:T13, "Command Timing"=w331:cluster{"Start Time (ms)":u32, "Iterations":i32})  [unwired: 9 in, 1 out]
        n160 = Unbundle(w331) -> ("Start Time (ms)"=w336:u32, "Iterations"=w333:i32)
        n161 = Unbundle(w332) -> ("Status"=w335:T1)  [unwired: 2 out]
        n162 = Subtract(x=w338, y=w336) -> (x-y=w337:u32)
        n163 = Bundle(w337, "Iterations"=w333) -> (w334:cluster{u32, "Iterations":i32})  [unwired: 1 in]
      }
      frame True {
        n164 = call "Drive Command Helper.vi"("Description"=w341, "SubSystem Data"=w340) -> ("Command Info Out"=w342:T13, "Command Timing"=w339:cluster{"Start Time (ms)":u32, "Iterations":i32})  [unwired: 7 in, 1 out]
        n165 = Unbundle(w342) -> ("Status"=w343:T1)  [unwired: 2 out]
      }
    }
    "Status" <- w327
    "Command Timing" <- w328
    n166 = global read "Drive Published Globals.vi" "DriveLastCommandStatus"() -> (→"DriveLastCommandStatus":T1)
    n167 = Wait (ms)(milliseconds to wait=u32 20) -> ()  [unwired: 1 out]
  }
